vi "SelectAcquisitionDirectoryforWrite-subvi.vi"(9 "Number of acquisition files":i32, 10 "Autostart?":bool, 11 "Acquisition directory root path":path=path "c:/scratch") -> (1 "OK?":bool=TRUE, 3 "Sequence files handle":T1)   [LabVIEW 2014]
uses:
  camera test/SubVIs/Initilize Globals.vi
panel:
  in  "Dummy refnum array":refnum<file>[](array[refnum])
  in  "Go?":bool
  in  "stop":bool
  in  "Digitize to new directory":path
  in  "Over-write exisitng:":path
  in  "New":bool=TRUE
  in  "Over-write":bool=TRUE
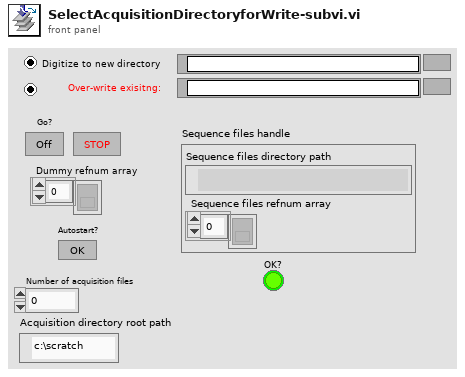
[diagram p1: front panel]
types:
  T1 = cluster{"Sequence files directory path":path, "Sequence files refnum array":refnum<file>[]}
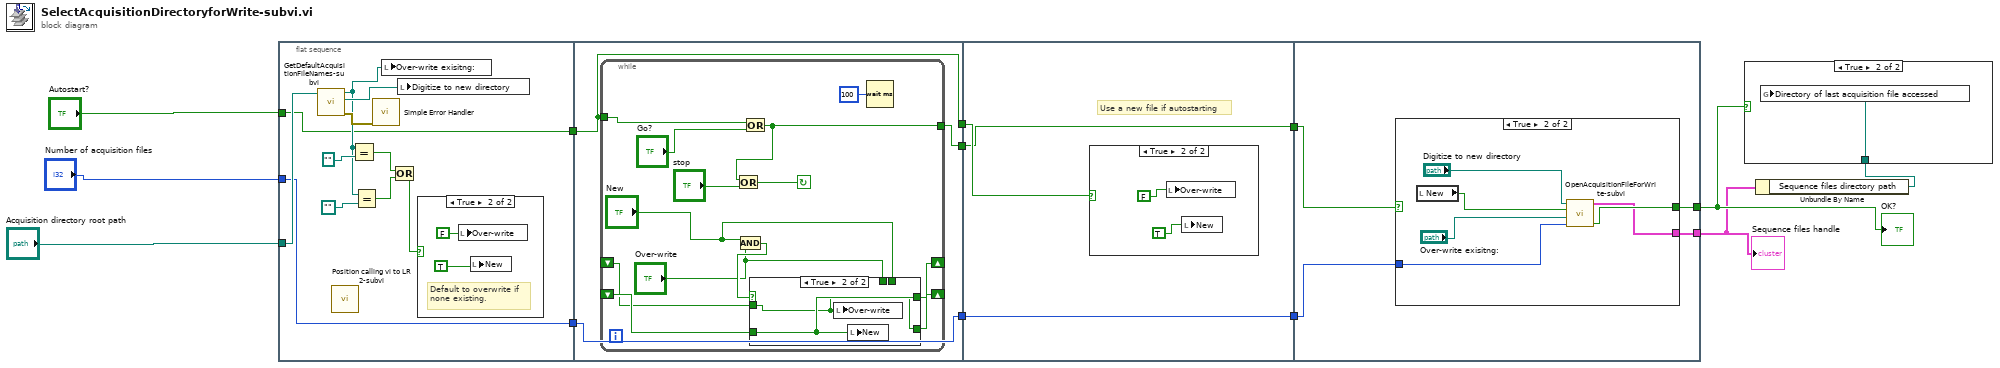
[diagram p0: block diagram]
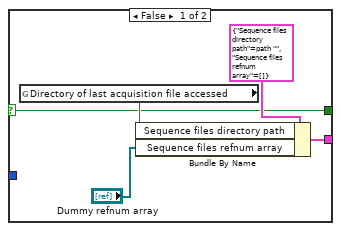
[diagram p6: hidden frame]
diagram:
  n1 = flat-sequence {
    tunnel: "Acquisition directory root path" -> [w20]
    tunnel: "Number of acquisition files" -> [w18]
    tunnel: "Autostart?" -> [w14]
    tunnel: [w18] -> w10
    tunnel: [w14] -> w9
    tunnel: w10 -> [w29]
    tunnel: w9 -> [w28]
    tunnel: [w29] -> w8
    tunnel: [w28] -> w7
    tunnel: [w27] -> w6
    tunnel: w8 -> [w49]
    tunnel: w7 -> [w48]
    tunnel: w6 -> [w47]
    tunnel: [w49] -> w5
    tunnel: [w47] -> w4
    tunnel: w5 -> [w55]
    tunnel: w4 -> [w54]
    tunnel: [w53] -> w3
    tunnel: [w52] -> w2
    frame #0 {
      n2 = call "GetDefaultAcquisitionFileNames-subvi.vi"("RAID root path"=w20) -> ("last directory path"=w15:path, "next directory path"=w16:path, "Error Out"=w17:errorcluster)  [unwired: 2 in, 1 out]
      n3 = call "Position calling vi to LR 2-subvi.vi"() -> ()  [unwired: 4 in, 2 out]
      n4 = Equal?(x=w15, y=path "") -> (x = y?=w21:bool)
      n5 = Equal?(x=w15, y=path "") -> (x = y?=w22:bool)
      n6 = call <vilib>:"Simple Error Handler.vi"("error in (no error)"=w17) -> ()  [unwired: 1 in, 8 out]
      n7 = local write "Over-write exisitng:"(w15) -> ()
      n8 = Or(x=w21, y=w22) -> (x .or. y?=w19:bool)
      n9 = local write "Digitize to new directory"(w16) -> ()
      n10 = case shown="True" w19 {
        frame False {
        }
        frame True {
          # "Default to overwrite if\nnone existing."
          n11 = local write "Over-write"(FALSE) -> ()
          n12 = local write "New"(TRUE) -> ()
        }
      }
    }
    frame #1 {
      n13 = while {
        tunnel: w28 -> [w42]
        tunnel: [w38] -> w27
        shift-right: [w30] -> _
        shift-left: _ -> [w32]
        shift-right: [w31] -> _
        shift-left: _ -> [w33]
        stop <- w37 continue-if-true
        n14 = And(x="New", y="Over-write") -> (x .and. y?=w36:bool)
        n15 = Or(x=w42, y="Go?") -> (x .or. y?=w38:bool)
        n16 = Or(x=w38, y="stop") -> (x .or. y?=w37:bool)
        n17 = case shown="True" w36 {
          tunnel: "Over-write" -> [w43 _]
          tunnel: "New" -> [w44 _]
          tunnel: w33 -> [_ w46]
          tunnel: [w44 w46] -> w30
          tunnel: w32 -> [_ w45]
          tunnel: [w43 w45] -> w31
          frame False {
          }
          frame True {
            n18 = local write "Over-write"(w45) -> ()
            n19 = local write "New"(w46) -> ()
          }
        }
        n20 = Wait (ms)(milliseconds to wait=u32 100) -> ()  [unwired: 1 out]
      }
    }
    frame #2 {
      # "Use a new file if autostarting"
      n21 = case shown="True" w48 {
        frame False {
        }
        frame True {
          n22 = local write "Over-write"(FALSE) -> ()
          n23 = local write "New"(TRUE) -> ()
        }
      }
    }
    frame #3 {
      n24 = case shown="True" w54 {
        selector: w54 -> [w57 _]
        tunnel: w55 -> [_ w61]
        tunnel: [w57 w66] -> w53
        tunnel: [w56 w65] -> w52
        frame False {
          n25 = global read "Initilize Globals.vi" "Directory of last acquisition file accessed"() -> (w60:path)
          n26 = Bundle By Name(cluster=T1 {"Sequence files directory path"=path "", "Sequence files refnum array"=[]} ("Sequence files handle"), "Sequence files directory path"=w60, "Sequence files refnum array"="Dummy refnum array") -> (w56:T1)
        }
        frame True {
          n27 = local read "New"() -> (w64:bool)
          n28 = call "OpenAcquisitionFileForWrite-subvi.vi"("Number of acquisition files"=w61, "Existing directory to over-write"="Over-write exisitng:", "Use new?"=w64, "New directory to create"="Digitize to new directory") -> ("OK?"=w66:bool, "Sequence files handle"=w65:T1)  [unwired: 6 in]
        }
      }
    }
  }
  n29 = Unbundle By Name(w2) -> ("Sequence files directory path"=w1:path)
  n30 = case shown="True" w3 {
    tunnel: w1 -> [_ w67]
    frame False {
    }
    frame True {
      n31 = global write "Initilize Globals.vi" "Directory of last acquisition file accessed"(w67) -> ()
    }
  }
  "OK?" <- w3
  "Sequence files handle" <- w2
